vi "GetInitialControlValues.vi"(8 "error in (no error)":errorcluster, 11 "UI_Interaction_Manager in":refnum<class "UI_Interaction_Manager.lvclass">) -> (0 "error out":errorcluster, 2 "ControlValueUpdates[]":T1[](array[typedef]), 3 "UI_Interaction_Manager out":refnum<class "UI_Interaction_Manager.lvclass">)   [LabVIEW 2011, in "UI_Interaction_Manager.lvclass"]
uses:
  UI_Interaction_Manager.lvclass
  TypeDefs/ControlValueUpdate.ctl
  UI_Interaction_Manager.lvclass/UI_Interaction_Manager.ctl
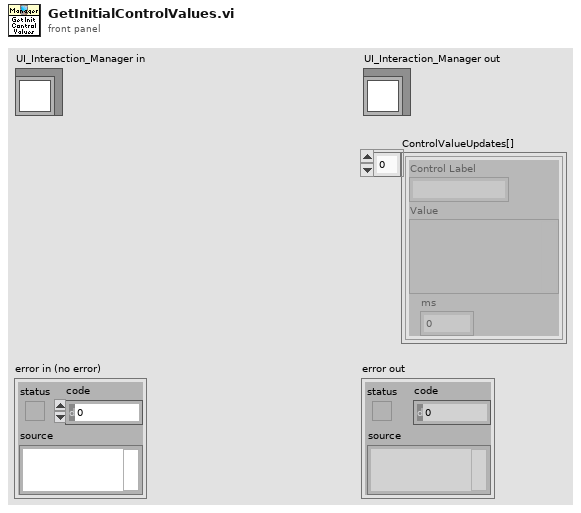
[diagram p1: front panel]
types:
  T1 = typedef "UI_Interaction_Manager.lvclass/ControlValueUpdate.ctl" = cluster{"Control Label":string, "Value":variant, "ms":u32}
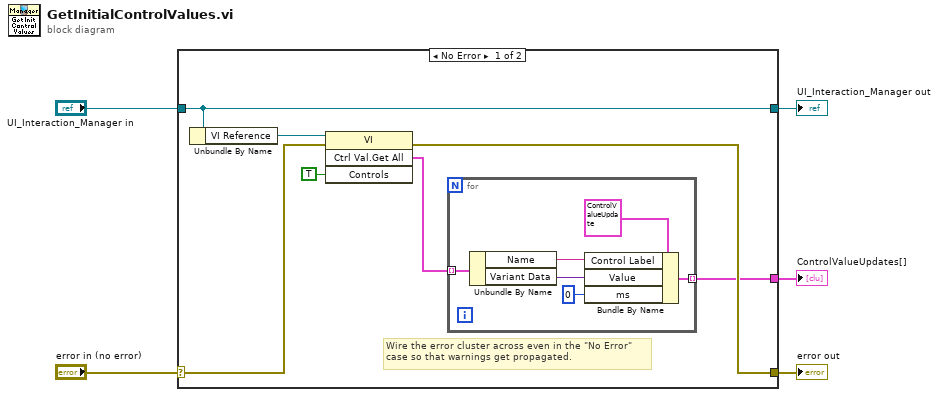
[diagram p0: block diagram]
diagram:
  n1 = case shown="No Error" "error in (no error)" {
    selector: "error in (no error)" -> [w8 w20]
    tunnel: [w7 w20] -> w4
    tunnel: [w10 w19] -> w2
    tunnel: "UI_Interaction_Manager in" -> [w10 w19]
    tunnel: [w6 _] -> w1
    frame No Error {
      # "Wire the error cluster across even in the \"No Error\"\ncase so that warnings get propagated."
      n2 = Unbundle By Name(w10) -> ("VI Reference"=w9:refnum<vi>)
      n3 = invoke class="VI" method="Ctrl Val.Get All"(reference=w9, error in=w8, "Controls"=TRUE) -> (error out=w7:errorcluster, "Get All Control Values Variant"=w11:cluster{"Name":string, "Variant Data":variant}[])  [unwired: 1 in, 2 out]
      n4 = for {
        tunnel: w11 -> [w18] mode=indexing
        tunnel: [w14] -> w6 mode=indexing
        n5 = Unbundle By Name(w18) -> ("Name"=w17:string, "Variant Data"=w16:variant)
        n6 = Bundle By Name(cluster=T1 {"Control Label"="", "Value"=variant, "ms"=0} ("Cluster"), "Control Label"=w17, "Value"=w16, "ms"=u32 0) -> (w14:T1)
      }
    }
    frame Error {
    }
  }
  "error out" <- w4
  "UI_Interaction_Manager out" <- w2
  "ControlValueUpdates[]" <- w1
